vi "tests.vi"   [LabVIEW 2012]
doc: "Statmach.vi is a state machine that can be ran from a Browser. The user can select on of five test to be ran by clicking on a corresponding link. Once the test completes the test's front panel is displayed on the Browser."
uses:
  <vilib>/addons/internet/NI_InternetTK_Core_VIs.lvlib
types:
  T1 = typedef "CGI Connection Info.ctl" = cluster{"name":string, "type":T2, "session":T3}
  T2 = typedef "CGI Request Type.ctl" = enum16{"cgi", ".spool first", ".spool", ".spool last"}
  T3 = typedef "HTTP Session.ctl" = refnum<k1>
  T4 = typedef "NI_FTP.lvlib/Keyed Array.ctl" = cluster{"keys":string[], "values":string[]}
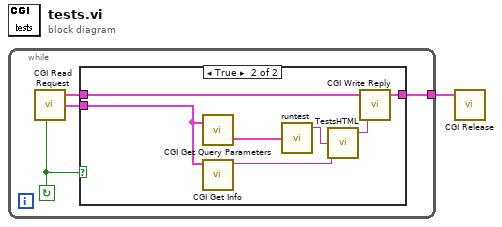
[diagram p0: block diagram]
diagram:
  n1 = while {
    tunnel: [w4] -> w1
    stop <- w3 continue-if-true
    n2 = call <vilib>:"CGI Read Request.vi"() -> ("valid request?"=w3:bool, "cgi connection info"=w5:T1, "env"=w2:T4)  [unwired: 4 in, 1 out]
    n3 = case shown="True" w3 {
      tunnel: [w6 w13] -> w4
      tunnel: w5 -> [w6 w12]
      tunnel: w2 -> [_ w8]
      frame False {
      }
      frame True {
        n4 = call <vilib>:"CGI Get Query Parameters.vi"("env"=w8) -> ("query params"=w9:T4)  [unwired: 2 out]
        n5 = call <vilib>:"CGI Get Info.vi"("env"=w8) -> ("cgi name"=w7:string)  [unwired: 4 in, 2 out]
        n6 = call "runtest.vi"("request"=w9) -> ("HTML out"=w10:string)  [unwired: 8 in]
        n7 = call "TestsHTML.vi"("Test HTML"=w10, "script name"=w7) -> ("HTML out"=w11:string)  [unwired: 7 in]
        n8 = call <vilib>:"CGI Write Reply.vi"("content"=w11, "cgi connection info"=w12) -> ("cgi connection info out"=w13:T1)  [unwired: 3 in]
      }
    }
  }
  n9 = call <vilib>:"CGI Release.vi"("cgi connection info"=w1) -> ()  [unwired: 5 in]
